vi "AIT 664 - Create Database Parmeters from Sysdef Tree.vi"(0 "Device Ptr":u64, 5 "664 Device":T1, 11 "error in":errorcluster) -> (6 "664 Device":T1, 15 "error out":errorcluster)   [LabVIEW 2013, in "AIT 664 Custom Device.lvlib"]
doc: "Extract system parameters from system configuration and match them up with configuraiton file"
uses:
  Controls/664 - XML Device Description.ctl
  Controls/664 - XML End System Description.ctl
  Controls/664 - XML Output VL.ctl
  Controls/664 - XML Tx Message Port.ctl
  Controls/664 - Sampling Type.ctl
  Controls/664 -Param.ctl
  Controls/664 - XML Input VL.ctl
  Controls/664 - XML Rx Message Port.ctl
  Controls and Global/Global.vi
  <vilib>/NI Veristand/Custom Device API/Get Item Property (String).vi
  <vilib>/NI Veristand/Custom Device Tools/Custom Device Utility Library/NI VeriStand - Search for All Items by GUID.vi
  <vilib>/NI Veristand/Custom Device API/Get Item Property (U32).vi
  AIT 664 Custom Device.lvlib
  <vilib>/NI Veristand/Custom Device Tools/Custom Device Utility Library/Custom Device Utility Library.lvlib
  <vilib>/NI Veristand/Custom Device API/Custom Device API.lvlib
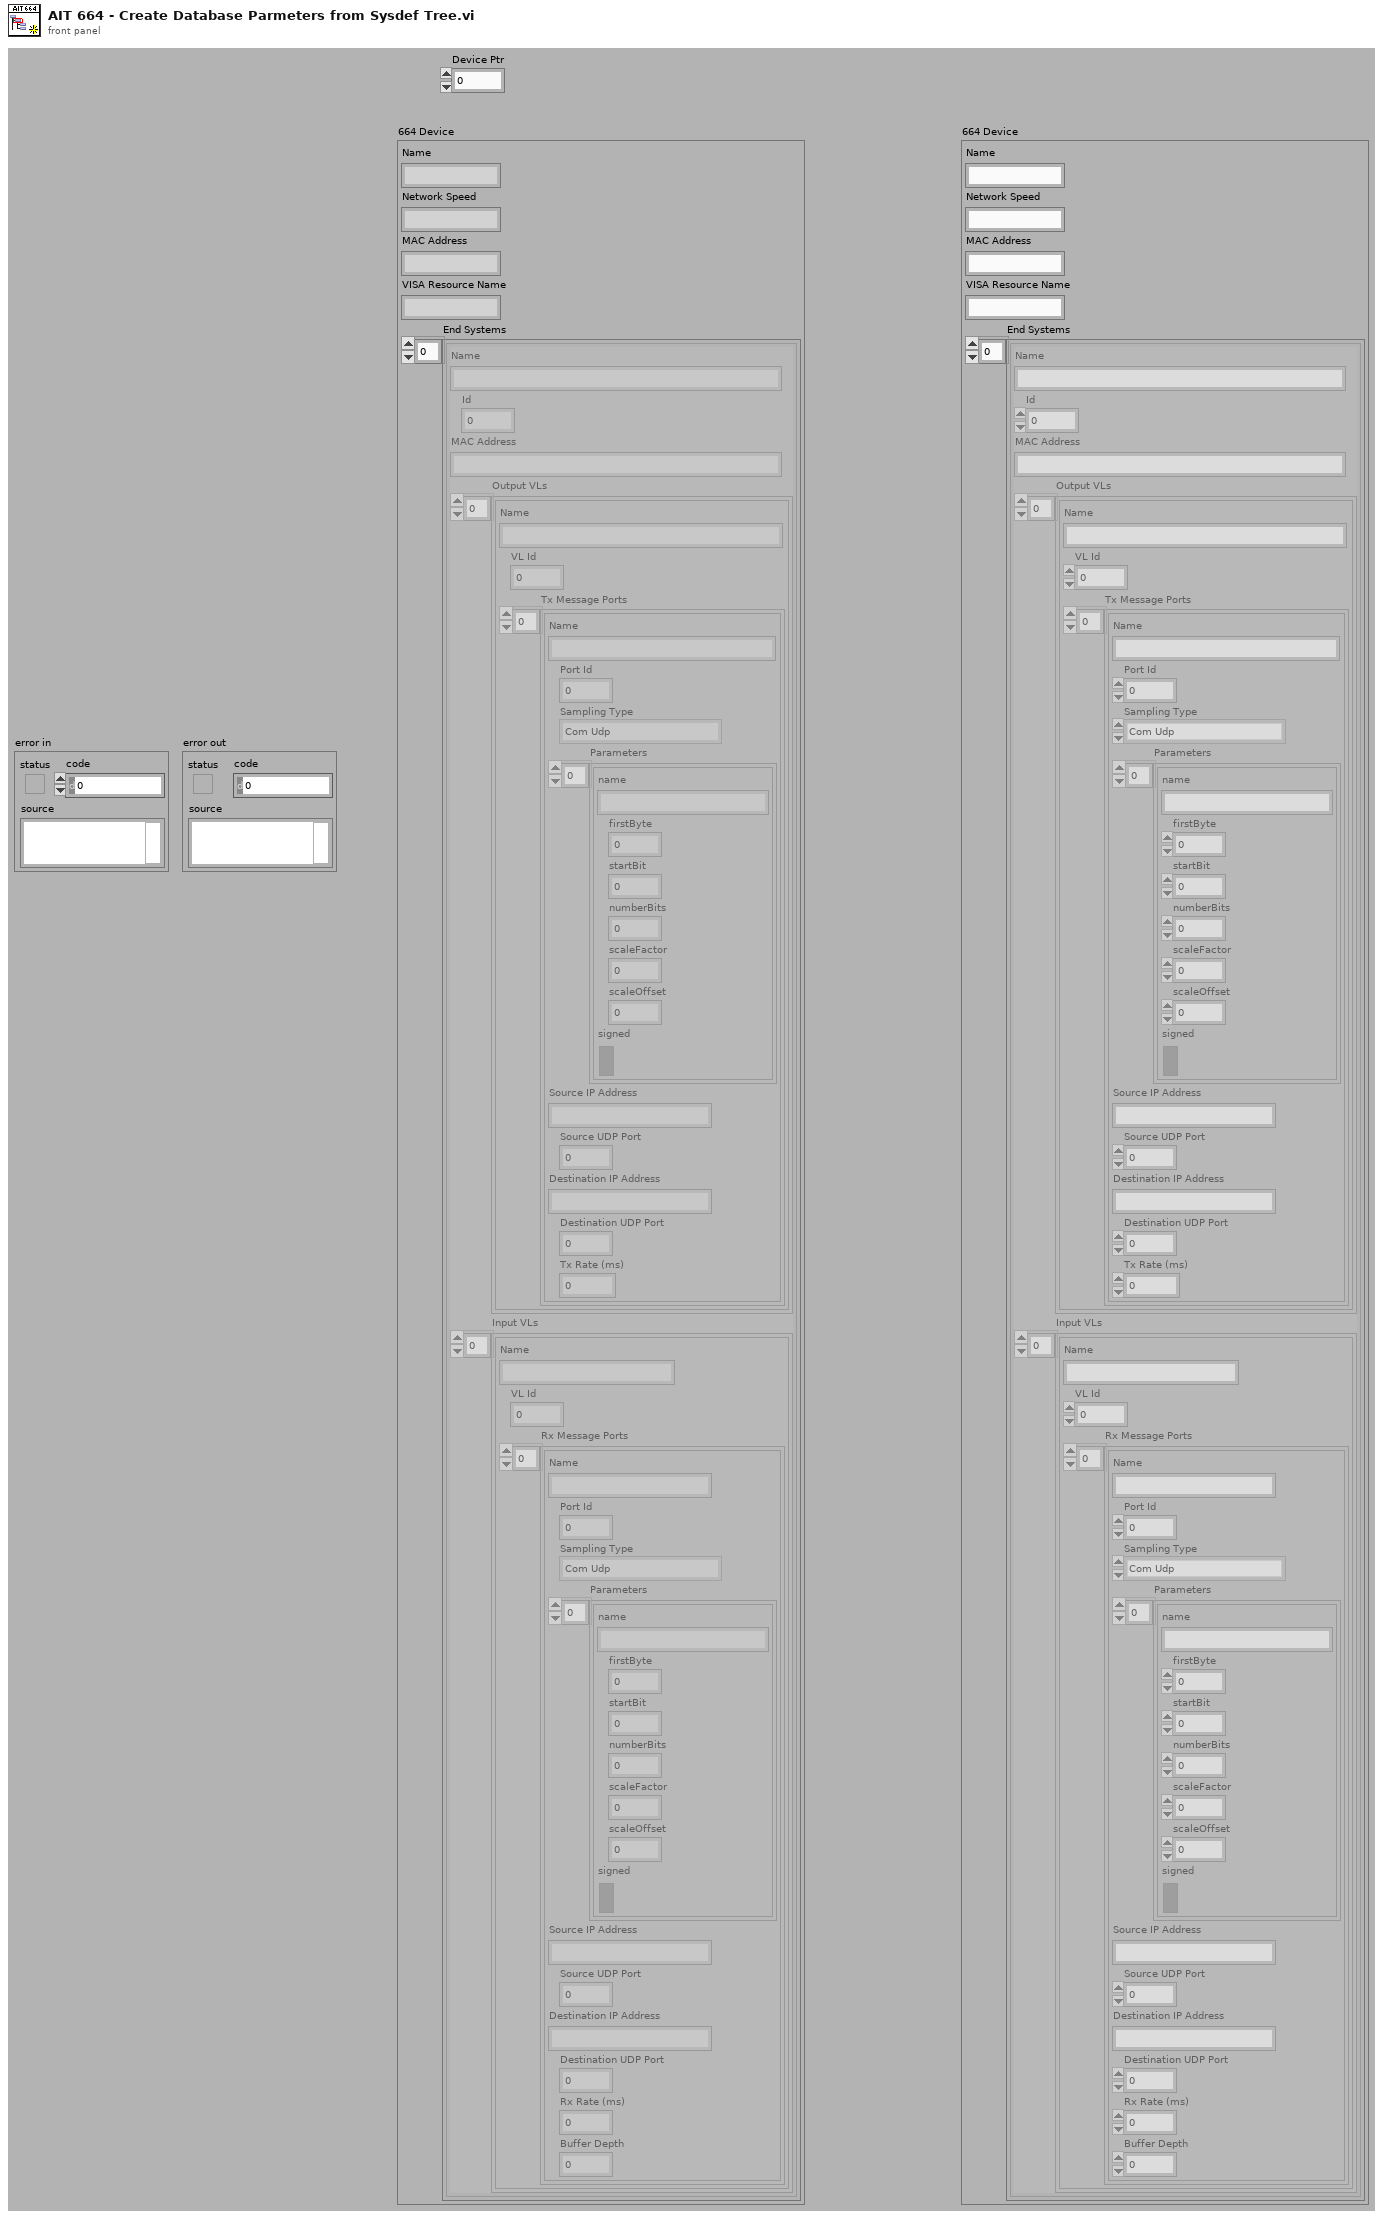
[diagram p1: front panel]
types:
  T1 = typedef "AIT 664 Custom Device.lvlib/664 - XML Device Description.ctl" = cluster{"Name":string, "Network Speed":string, "MAC Address":string, "VISA Resource Name":string, "End Systems":T2[]}
  T2 = typedef "AIT 664 Custom Device.lvlib/664 - XML End System Description.ctl" = cluster{"Name":string, "Id":u32, "MAC Address":string, "Output VLs":T3[], "Input VLs":T7[]}
  T3 = typedef "AIT 664 Custom Device.lvlib/664 - XML Output VL.ctl" = cluster{"Name":string, "VL Id":u32, "Tx Message Ports":T4[]}
  T4 = typedef "AIT 664 Custom Device.lvlib/664 - XML Tx Message Port.ctl" = cluster{"Name":string, "Port Id":u32, "Sampling Type":T5, "Parameters":T6[], "Source IP Address":string, "Source UDP Port":u32, "Destination IP Address":string, "Destination UDP Port":u32, "Tx Rate (ms)":u32}
  T5 = typedef "AIT 664 Custom Device.lvlib/664 - Sampling Type.ctl" = enum16{"Com Udp", "Com Udp Queuing", "Sap Udp", "Sap Ip", "Sap Mac", "Unknown"}
  T6 = typedef "AIT 664 Custom Device.lvlib/664 -Param.ctl" = cluster{"name":string, "firstByte":i32, "startBit":i32, "numberBits":i32, "scaleFactor":dbl, "scaleOffset":dbl, "signed":bool}
  T7 = typedef "AIT 664 Custom Device.lvlib/664 - XML Input VL.ctl" = cluster{"Name":string, "VL Id":u32, "Rx Message Ports":T8[]}
  T8 = typedef "AIT 664 Custom Device.lvlib/664 - XML Rx Message Port.ctl" = cluster{"Name":string, "Port Id":u32, "Sampling Type":T5, "Parameters":T6[], "Source IP Address":string, "Source UDP Port":u32, "Destination IP Address":string, "Destination UDP Port":u32, "Rx Rate (ms)":u32, "Buffer Depth":u32}
  T9 = typedef "Custom Device API.lvlib/Custom Device Item Ref.ctl" = u64
  T10 = typedef "Custom Device API.lvlib/Custom Device Item Info.ctl" = cluster{"Name":string, "Is Channel":bool, "GUID":string, "Is Waveform":bool}
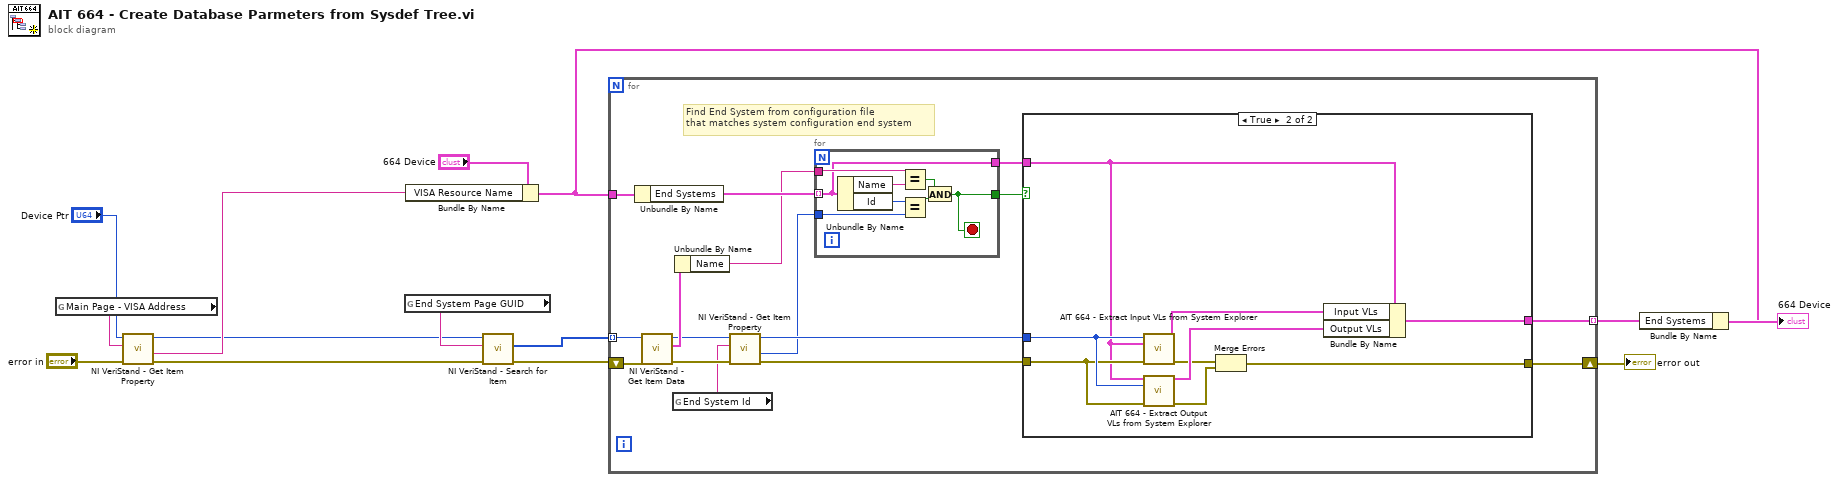
[diagram p0: block diagram]
diagram:
  n1 = global read "Global.vi" "Main Page - VISA Address"() -> (w4:string)
  n2 = call-poly <vilib>:"NI VeriStand - Get Item Property.vi"("error in (no error)"="error in", "Property Name"=w4, "Item Ref in"="Device Ptr") -> ("error out"=w2:errorcluster, "Value"=w3:string, "Item Ref out"=w1:T9)  [unwired: 5 in, 1 out]
  n3 = global read "Global.vi" "End System Page GUID"() -> (w14:string)
  n4 = Bundle By Name(cluster="664 Device", "VISA Resource Name"=w3) -> (w7:T1)
  n5 = call-poly <vilib>:"NI VeriStand - Search for Item.vi"("error in"=w2, "Item GUID"=w14, "Section Ref in"=w1) -> ("error out"=w10:errorcluster, "Item Refs"=w13:T9[])  [unwired: 5 in, 2 out]
  n6 = for {
    tunnel: w13 -> [w26] mode=indexing
    tunnel: w7 -> [w23]
    tunnel: [w17] -> w12 mode=indexing
    shift-right: [w16] -> w9
    shift-left: w10 -> [w15]
    # "Find End System from configuration file\nthat matches system configuration end system"
    n7 = Unbundle By Name(w23) -> ("End Systems"=w22:T2[])
    n8 = call <vilib>:"NI VeriStand - Get Item Data.vi"("error in (no error)"=w15, "Item Ref in"=w26) -> ("error out"=w28:errorcluster, "Item Info"=w30:T10, "Item Ref out"=w29:T9)  [unwired: 6 in, 1 out]
    n9 = global read "Global.vi" "End System Id"() -> (w27:string)
    n10 = Unbundle By Name(w30) -> ("Name"=w21:string)
    n11 = call-poly <vilib>:"NI VeriStand - Get Item Property.vi"("error in (no error)"=w28, "Property Name"=w27, "Item Ref in"=w29) -> ("error out"=w25:errorcluster, "Value"=w20:u32, "Item Ref out"=w24:T9)  [unwired: 5 in, 1 out]
    n12 = for {
      tunnel: w22 -> [w41] mode=indexing
      tunnel: w21 -> [w45]
      tunnel: w20 -> [w47]
      tunnel: [w42] -> w19
      tunnel: [w41] -> w18
      stop <- w42 stop-if-true
      n13 = Unbundle By Name(w41) -> ("Name"=w46:string, "Id"=w48:u32)
      n14 = Equal?(x=w45, y=w46) -> (x = y?=w44:bool)
      n15 = Equal?(x=w48, y=w47) -> (x = y?=w43:bool)
      n16 = And(x=w44, y=w43) -> (x .and. y?=w42:bool)
    }
    n17 = case shown="True" w19 {
      tunnel: w25 -> [w31 w37]
      tunnel: w24 -> [_ w38]
      tunnel: w18 -> [_ w36]
      tunnel: [_ w39] -> w17
      tunnel: [w31 w32] -> w16
      frame False {
      }
      frame True {
        n18 = call "AIT 664 - Extract Input VLs from System Explorer.vi"("Item Ref"=w38, "664 End System"=w36, "error in (no error)"=w37) -> ("Input VLs Out"=w35:T7[], "error out"=w34:errorcluster)  [unwired: 11 in]
        n19 = call "AIT 664 - Extract Output VLs from System Explorer.vi"("664 End System"=w36, "Item Ref in"=w38, "error in (no error)"=w37) -> ("Output VLs out"=w40:T3[], "error out"=w33:errorcluster)  [unwired: 11 in]
        n20 = Merge Errors(w34, w33) -> (w32:errorcluster)
        n21 = Bundle By Name(cluster=w36, "Input VLs"=w35, "Output VLs"=w40) -> (w39:T2)
      }
    }
  }
  "error out" <- w9
  n22 = Bundle By Name(cluster=w7, "End Systems"=w12) -> (→"664 Device":T1)
